vi "PanelFactory.vi"(8 "error in (no error)":errorcluster, 10 "ThreadName(\"\")":string, 11 "User_Actor in":refnum<class "User_Actor.lvclass">) -> (0 "error out":errorcluster, 2 "MemberPanel(Product)":refnum<class "MemberPanel.lvclass">, 3 "User_Actor out":refnum<class "User_Actor.lvclass">)   [LabVIEW 2015, in "User_Actor.lvlib" / "User_Actor.lvclass"]
uses:
  User_Actor.lvclass
  Member_Actor/MemberPanel/MemberPanel.lvclass
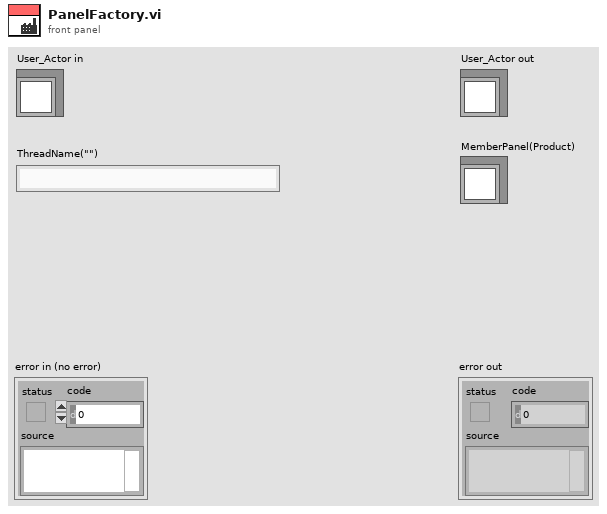
[diagram p1: front panel]
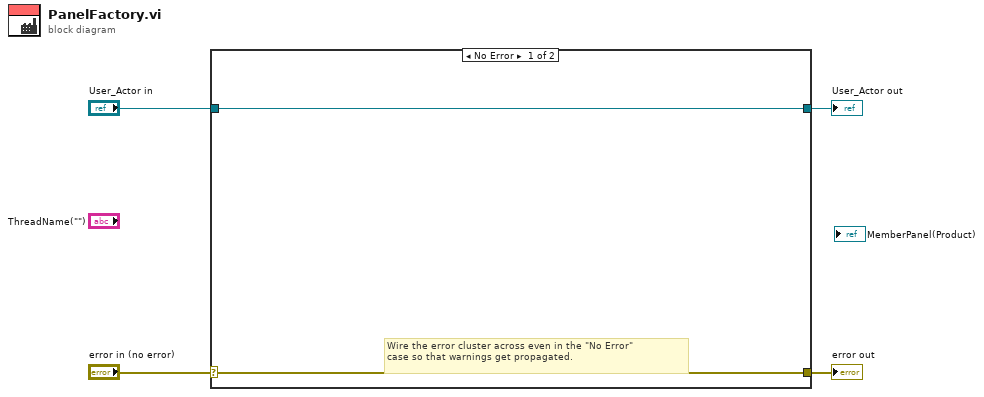
[diagram p0: block diagram]
diagram:
  n1 = case shown="No Error" "error in (no error)" {
    selector: "error in (no error)" -> [w5 w8]
    tunnel: [w5 w8] -> w3
    tunnel: [w6 w7] -> w1
    tunnel: "User_Actor in" -> [w6 w7]
    frame No Error {
      # "Wire the error cluster across even in the \"No Error\"\ncase so that warnings get propagated."
    }
    frame Error {
    }
  }
  "error out" <- w3
  "User_Actor out" <- w1
